vi "Collect XYZ piezo metadata.vi"(0 "reference in":refnum<class "metadata.lvclass">, 5 "error in (no error)":errorcluster) -> (14 "reference out":refnum<class "metadata.lvclass">, 16 "Metadata":T1, 19 "error out":errorcluster)   [LabVIEW 2019, in "metadata.lvclass"]
uses:
  metadata.lvclass
  Metadata output --cluster.ctl
panel:
  out "List property names":string
  out "Property Names":string[](array[string])
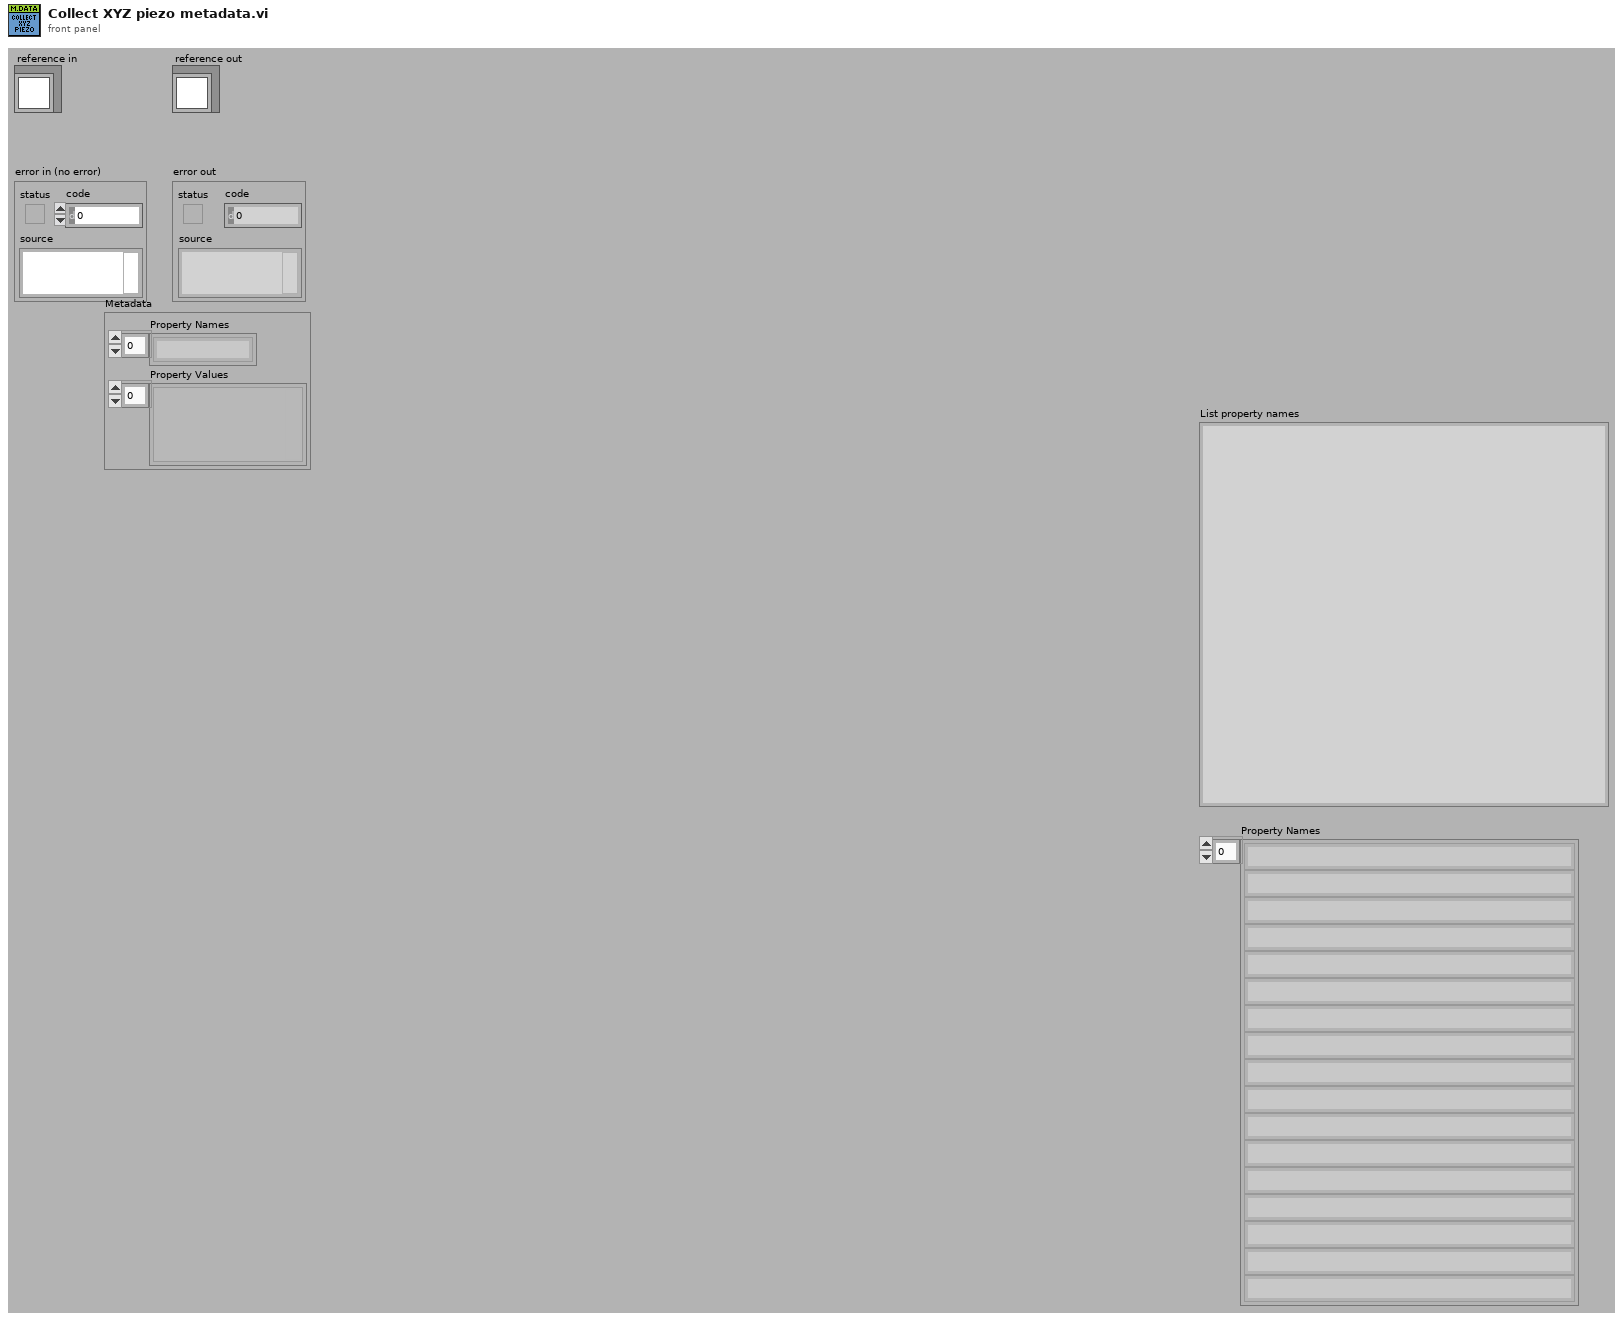
[diagram p1: front panel]
types:
  T1 = typedef "metadata.lvclass/Metadata output --cluster.ctl" = cluster{"Property Names":string[], "Property Values":variant[]}
  T2 = typedef "metadata.lvclass/ObjectAttributes.ctl" = cluster{"MyAttribute":dbl, "System Control":T3, "file info":T4, "Sample info":T5, "Cantilever info":T6, "XYZ piezos":T7, "Mapping":T8, "Fcurve segment":T9[], "Fast fpga segment":T11, "Chirp":T12, "precision (6)":i16, "width (-)":i16, "Metadata":T1, "config filepath":path, "Section names []":string[], "Property names []":string[], "nb elements":u16}
  T3 = typedef "metadata.lvclass/System control parameters.ctl" = cluster{"FPGA SW version":string, "TDMS file version":string, "Instrument":string, "Instrument model":string, "Instrument scanner":string, "Instrument clockrate (Mhz)":string, "Instrument tick time (us)":string}
  T4 = typedef "metadata.lvclass/File info parameters.ctl" = cluster{"Time Stamp":timestamp, "Filename":string, "Filepath":path, "User":string, "Experiment_name":string, "Curve_id":string, "number_segments":u8, "number_consecutive_scans":u32}
  T5 = typedef "metadata.lvclass/Sample info parameters.ctl" = cluster{"Sample name":string, "Sample species":string}
  T6 = typedef "metadata.lvclass/Cantilever info parameters.ctl" = cluster{"spring constant calib method":string, "invOLS calib method":string, "thermal calib deflection channel":string, "model":string, "shape":string, "tip geometry":string, "Laser sum (V)":dbl, "Laser power (mA)":dbl, "invOLS_(nm/V)":dbl, "spring constant nominal (N/m)":dbl, "spring constant calib (N/m)":dbl, "resosnance frequency air calib (Hz)":dbl, "resosnance frequency calib (Hz)":dbl, "quality factor":dbl, "Acoefficident_GCI_(nN.s^1.3/m)":dbl, "half angle (deg)":dbl, "tip radius (m)":dbl, "tip height (m)":dbl, "system mount angle (deg)":dbl}
  T7 = typedef "metadata.lvclass/XYZ piezos parameters.ctl" = cluster{"X stage piezo sensitivity (nm/V)":dbl, "X stage piezo gain":dbl, "X velocity (V/tick)":dbl, "X closed loop":bool, "Y stage piezo sensitivity (nm/V)":dbl, "Y stage piezo gain":dbl, "Y velocity (V/tick)":dbl, "Y closed loop":bool, "Z stage piezo sensitivity (nm/V)":dbl, "Z stage piezo gain":dbl, "Z closed loop":bool, "X position (V)":dbl, "Y position (V)":dbl}
  T8 = typedef "metadata.lvclass/Mapping parameters.ctl" = cluster{"Mapping":bool, "index":u16, "position row":u16, "position column":u16, "next position row":i16, "next position column":i16, "X initial position (V)":dbl, "Y initial position (V)":dbl, "X step size (V)":dbl, "Y step size (V)":dbl}
  T9 = typedef "metadata.lvclass/Fcurve segment.ctl" = cluster{"type":T10, "fast_fpga_trigger":bool, "nb":u8, "duration (ticks)":i64, "nb points":i32, "sampling rate (S/s)":u32, "Zpiezo control out":string, "initial deflection (V)":dbl, "relative setpoint":bool, "setpoint on":bool, "setpoint (V)":dbl, "setpoint trigger channel":string, "velocity (V/tick)":dbl, "Z position setpoint trigger (V)":dbl, "Z retract length (V)":dbl, "dec factor":u32}
  T10 = typedef "metadata.lvclass/Segment type--combobox.ctl" = string
  T11 = typedef "metadata.lvclass/fast fpga segment parameters.ctl" = cluster{"Fast start time trigger":timestamp, "nb_points":u32, "sampling_rate_(S/s)":u32, "duration_(ticks)":u32}
  T12 = typedef "metadata.lvclass/Chirp added parameters.ctl" = cluster{"f start (Hz)":dbl, "f end (Hz)":dbl, "Sweep type":string}
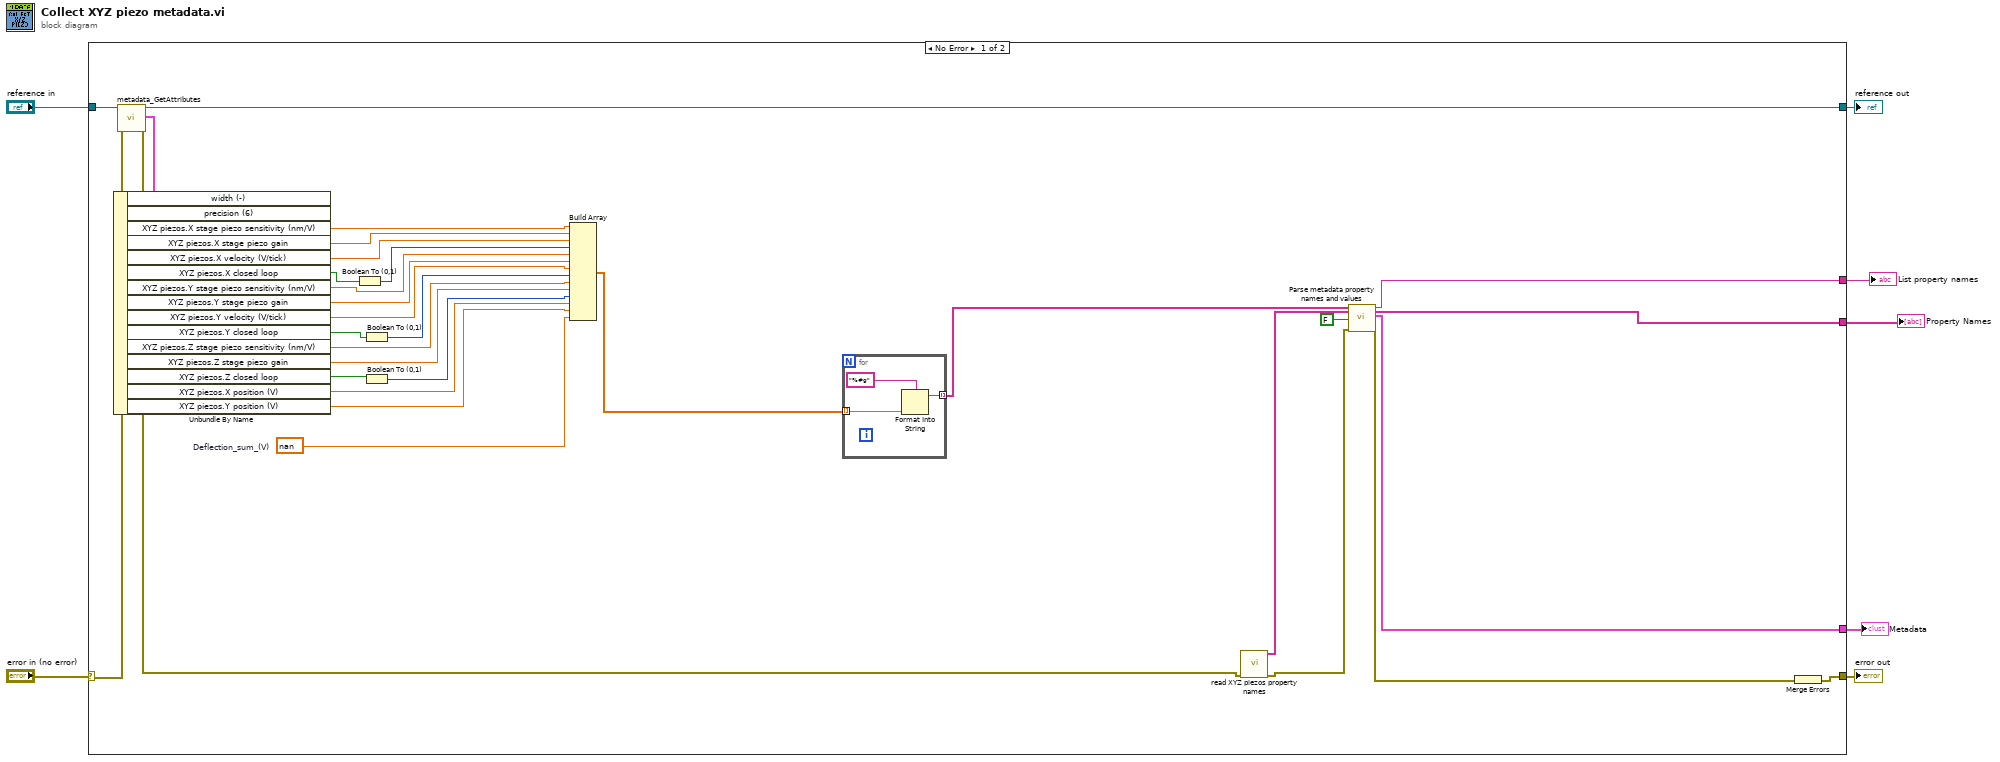
[diagram p0: block diagram]
diagram:
  n1 = case shown="No Error" "error in (no error)" {
    selector: "error in (no error)" -> [w36 w44]
    tunnel: [w39 w44] -> w6
    tunnel: [w37 w43] -> w4
    tunnel: "reference in" -> [w38 w43]
    tunnel: [w33 _] -> w3
    tunnel: [w32 _] -> w1
    tunnel: [w31 _] -> w2
    frame No Error {
      w8 = nan  # Deflection_sum_(V)
      n2 = call "metadata_GetAttributes.vi"("reference in"=w38, "error in (no error)"=w36) -> ("reference out"=w37:refnum<class "metadata.lvclass">, "attributes"=w35:T2, "error out"=w28:errorcluster)  [unwired: 14 in, 1 out]
      n3 = Unbundle By Name(w35) -> ("XYZ piezos.X stage piezo sensitivity (nm/V)"=w25:dbl, "XYZ piezos.X stage piezo gain"=w24:dbl, "XYZ piezos.X velocity (V/tick)"=w23:dbl, "XYZ piezos.X closed loop"=w22:bool, "XYZ piezos.Y stage piezo sensitivity (nm/V)"=w20:dbl, "XYZ piezos.Y stage piezo gain"=w19:dbl, "XYZ piezos.Y velocity (V/tick)"=w18:dbl, "XYZ piezos.Y closed loop"=w16:bool, "XYZ piezos.Z stage piezo sensitivity (nm/V)"=w15:dbl, "XYZ piezos.Z stage piezo gain"=w14:dbl, "XYZ piezos.Z closed loop"=w13:bool, "XYZ piezos.X position (V)"=w11:dbl, "XYZ piezos.Y position (V)"=w10:dbl)  [unwired: 2 out]
      n4 = Boolean To (0,1)(Boolean=w22) -> (0, 1=w21:i16)
      n5 = Boolean To (0,1)(Boolean=w16) -> (0, 1=w17:i16)
      n6 = Boolean To (0,1)(Boolean=w13) -> (0, 1=w12:i16)
      n7 = Build Array(w25, w24, w23, w21, w20, w19, w18, w17, w15, w14, w12, w11, w10, w8) -> (w9:dbl[])
      n8 = for {
        tunnel: [w41] -> w30 mode=indexing
        tunnel: w9 -> [w40] mode=indexing
        n9 = Format Into String(format string="%#g", w40) -> (resulting string=w41:string)  [unwired: 2 in, 1 out]
      }
      n10 = call "read XYZ piezos property names.vi"("error in (no error)"=w28) -> ("XYZ piezos"=w26:string[], "error out"=w27:errorcluster)  [unwired: 17 in]
      n11 = call "Parse metadata property names and values.vi"("Data intput []"=w30, "property names []"=w26, "List param"=FALSE, "error in (no error)"=w27) -> ("Param list"=w31:string, "Array"=w33:string[], "output cluster"=w32:T1, "error out"=w34:errorcluster)  [unwired: 12 in]
      n12 = Merge Errors(w34) -> (w39:errorcluster)
    }
    frame Error {
    }
  }
  "error out" <- w6
  "reference out" <- w4
  "Property Names" <- w3
  "List property names" <- w2
  "Metadata" <- w1
